vi "Overlay_NewlyIntegrated_SR.vi"(8 "error in (no error)":errorcluster, 10 "AlgoType array out":T1[](array[typedef]), 11 "Result data out 2":T2={"Measurement Names Array"=[], "Pass-Fail Array"=[], "Measurement Values Array "=[], "Roi for overlay (Arrows) Array"=[], "Algo Type Array"=[], "Image Array"=[], "Clamp operations"=enum."Average Clamp", "  Search Direction "=[], "Images_Array_in"=[], "ResultPF"=FALSE, "Total Cluster Values"={"Total Pass"=0.0, "Total Fail"=0.0, "Total Count"=0.0, "Total Pass-T"=0.0, "Total Pass-B"=0.0, "Total Fail-T"=0.0, "Total Fail-B"=0.0, "Total Count-T"=0.0, "Total Count-B"=0.0}, "Reel Counter Cluster"={"Reel Pass-T"=0.0, "Reel Pass-B"=0.0, "Reel Fail-T"=0.0, "Reel Fail-B"=0.0, "Reel Count-T"=0.0, "Reel Count-B"=0.0}, "Tolerance  Array"=[], "Array of Cam Spec Control Bool"=[], "Control Pass Fail Array"=[], "Specification Pass Fail Array"=[]}) -> (0 "error in (no error)":errorcluster)   [LabVIEW 2015, in "Algorithm.lvclass"]
uses:
  FrameworkOverrides/Algorithm.lvclass
  Controls/Result Cluster.ctl
  Controls/Algo_Type.ctl
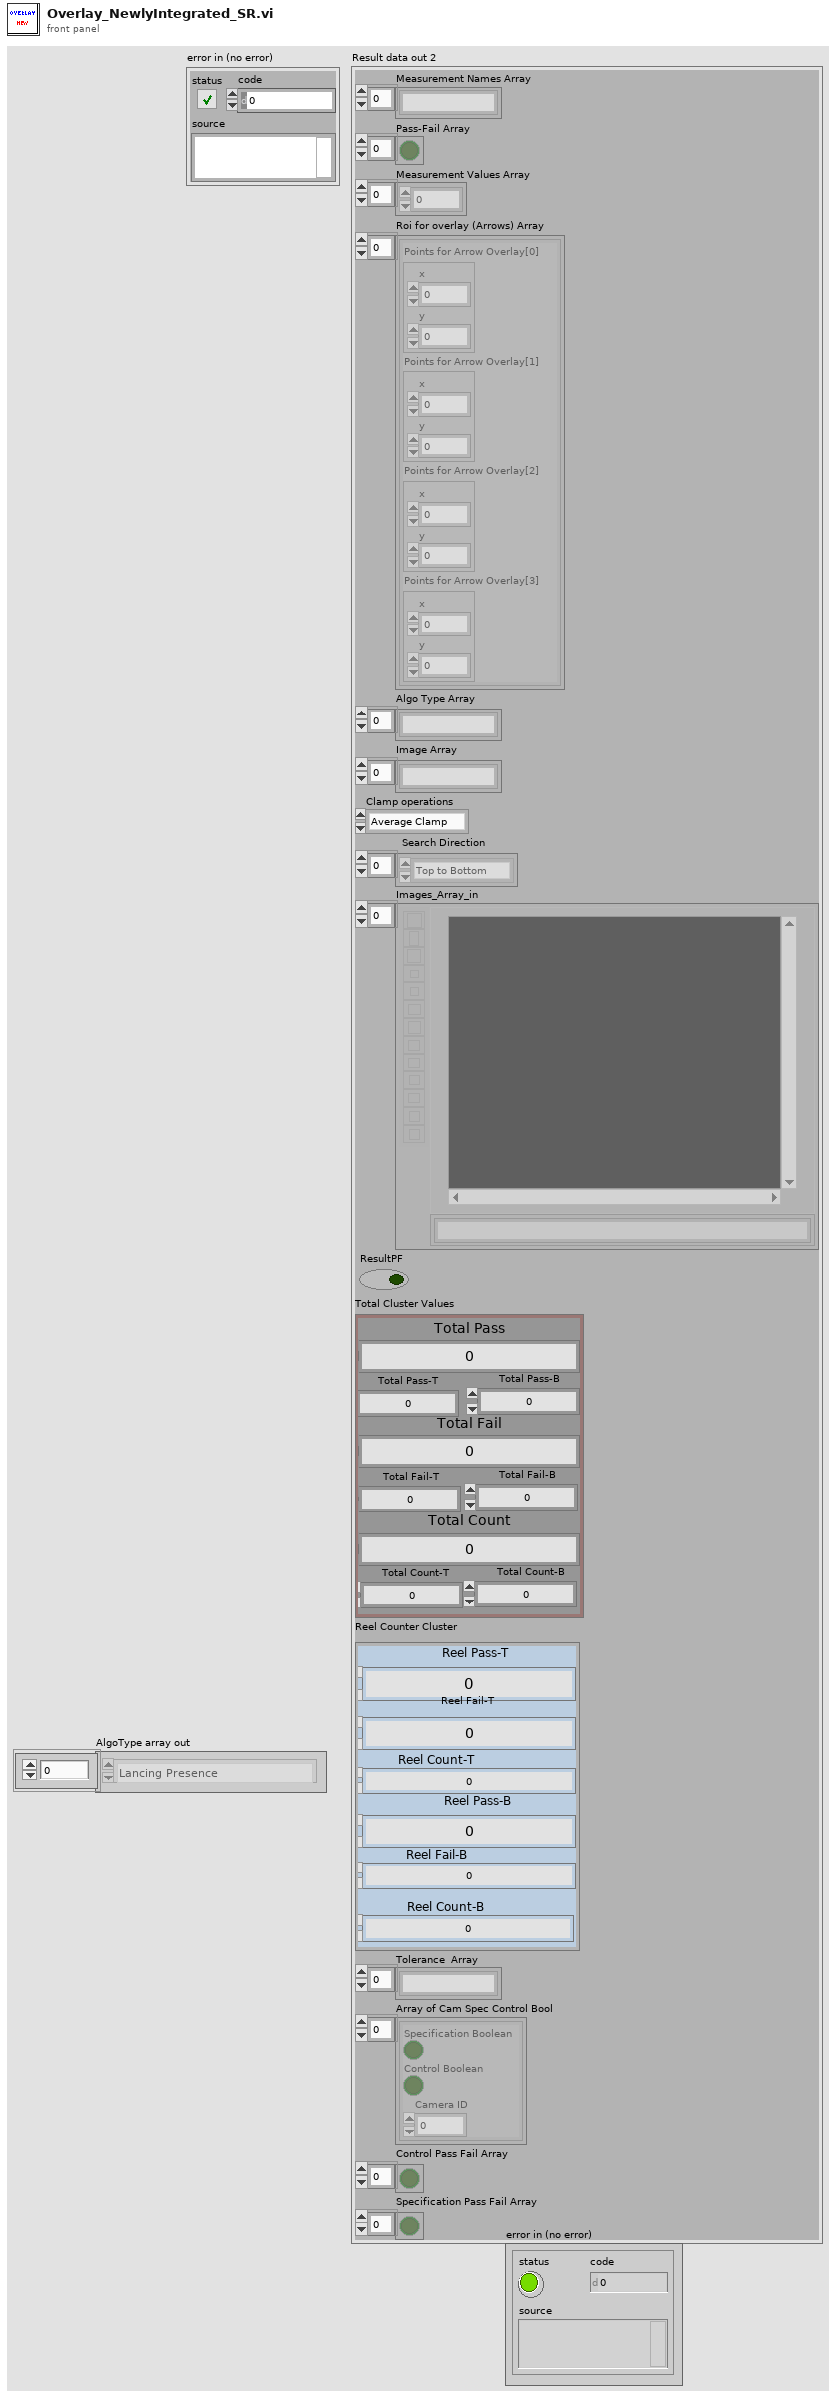
[diagram p1: front panel]
types:
  T1 = typedef "Algorithm.lvclass/Algo_Type.ctl" = enum16{"Lancing Presence", "Pitch", "Circlular_Dia", "LipGap", "Angle", "BarbHeight", "102 EON Presence", "102 Lipgap", "Lip Symmetry", "Lip Level", "Box Width", "Lip Outer Width", "EON Width", "EON Presence", "Lipgap FCI", "Linear", "Projected Distance_Type_1", " Projected Distance_Type_2", "Projected Distance_Type_3", "AET", "AET Min", "TT_Width", "Lancing", "WND", "Linear_Lenght1", "Linear_Lenght2", "Side_E", "Side_E1", "Top_E", "Edge Distance", "Side Vertical Minimum"}
  T2 = typedef "Algorithm.lvclass/Result Cluster.ctl" = cluster{"Measurement Names Array":string[], "Pass-Fail Array":bool[], "Measurement Values Array ":dbl[], "Roi for overlay (Arrows) Array":cluster{"Points for Arrow Overlay[0]":cluster{"x":dbl, "y":dbl}, "Points for Arrow Overlay[1]":cluster{"x":dbl, "y":dbl}, "Points for Arrow Overlay[2]":cluster{"x":dbl, "y":dbl}, "Points for Arrow Overlay[3]":cluster{"x":dbl, "y":dbl}}[], "Algo Type Array":string[], "Image Array":string[], "Clamp operations":enum16{"Min Clamp", "Max Clamp", "Average Clamp"}, "  Search Direction ":enum16{"Left to Right", "Right to Left", "Top to Bottom", "Bottom to Top"}[], "Images_Array_in":T3[], "ResultPF":bool, "Total Cluster Values":cluster{"Total Pass":dbl, "Total Fail":dbl, "Total Count":dbl, "Total Pass-T":dbl, "Total Pass-B":dbl, "Total Fail-T":dbl, "Total Fail-B":dbl, "Total Count-T":dbl, "Total Count-B":dbl}, "Reel Counter Cluster":cluster{"Reel Pass-T":dbl, "Reel Pass-B":dbl, "Reel Fail-T":dbl, "Reel Fail-B":dbl, "Reel Count-T":dbl, "Reel Count-B":dbl}, "Tolerance  Array":string[], "Array of Cam Spec Control Bool":cluster{"Specification Boolean":bool, "Control Boolean":bool, "Camera ID":i8}[], "Control Pass Fail Array":bool[], "Specification Pass Fail Array":bool[]}
  T3 = typedef "IMAQ Image.ctl" = refnum<image>
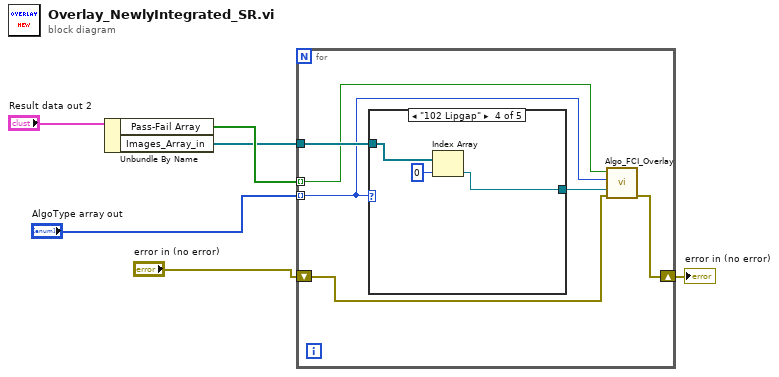
[diagram p0: block diagram]
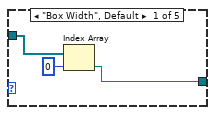
[diagram p2: hidden frame]
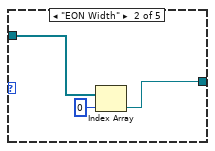
[diagram p3: hidden frame]
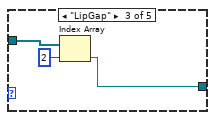
[diagram p4: hidden frame]
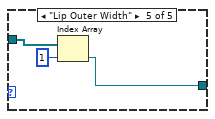
[diagram p5: hidden frame]
diagram:
  n1 = Unbundle By Name("Result data out 2") -> ("Pass-Fail Array"=w5:bool[], "Images_Array_in"=w3:T3[])
  n2 = for {
    tunnel: w5 -> [w11] mode=indexing
    tunnel: "AlgoType array out" -> [w10] mode=indexing
    tunnel: w3 -> [w12]
    shift-right: [w7] -> w1
    shift-left: "error in (no error)" -> [w8]
    n3 = case shown="\"102 Lipgap\"" w10 {
      tunnel: w12 -> [w15 w18 w21 w24 w27]
      tunnel: [w14 w16 w19 w22 w26] -> w9
      frame "Box Width", Default {
        n4 = Index Array(array=w15, index=0) -> (element=w14:T3)
      }
      frame "EON Width" {
        n5 = Index Array(array=w18, index=0) -> (element=w16:T3)
      }
      frame "LipGap" {
        n6 = Index Array(array=w21, index=2) -> (element=w19:T3)
      }
      frame "102 Lipgap" {
        n7 = Index Array(array=w24, index=0) -> (element=w22:T3)
      }
      frame "Lip Outer Width" {
        n8 = Index Array(array=w27, index=1) -> (element=w26:T3)
      }
    }
    n9 = call "Algo_FCI_Overlay.vi"("error in (no error)"=w8, "Image in"=w9, "Algo Type"=w10, "Enabled?"=w11) -> ("error out"=w7:errorcluster)  [unwired: 7 in]
  }
  "error in (no error)" <- w1
